vi "Display Album Library.vi"(8 "error in (no error)":errorcluster, 10 "MusicLibrary":refnum<class "MusicLibrary.lvclass">, 11 "SongBrowserActor in":refnum<class "SongBrowserActor.lvclass">) -> (0 "error out":errorcluster, 3 "SongBrowserActor out":refnum<class "SongBrowserActor.lvclass">)   [LabVIEW 2015, in "SongBrowserActor.lvlib" / "SongBrowserActor.lvclass"]
uses:
  SongBrowserActor.lvclass
  file/MusicElement/MusicElementLibrary/MusicLibrary/MusicLibrary.lvclass
  SongBrowserActor.lvclass/SongBrowserActor.ctl
  builds/xctls/Album Browser/Album Browser.lvlibp/app/xctls/Album Browser/Album Browser/Album Browser.xctl
  file/MusicElement/MusicElementLibrary/MusicElementLibrary.lvclass
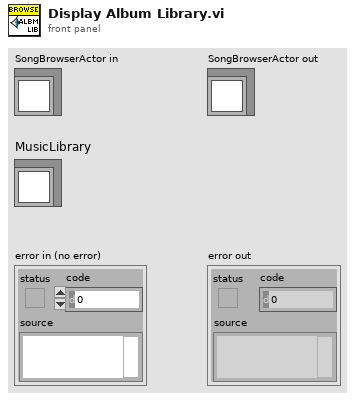
[diagram p1: front panel]
types:
  T1 = typedef "Music Library Element Display.ctl" = cluster{"Name":string, "Details":string, "Duration (s)":T2, "Click":bool}
  T2 = typedef "Song.lvclass/Song Duration.ctl" = timestamp
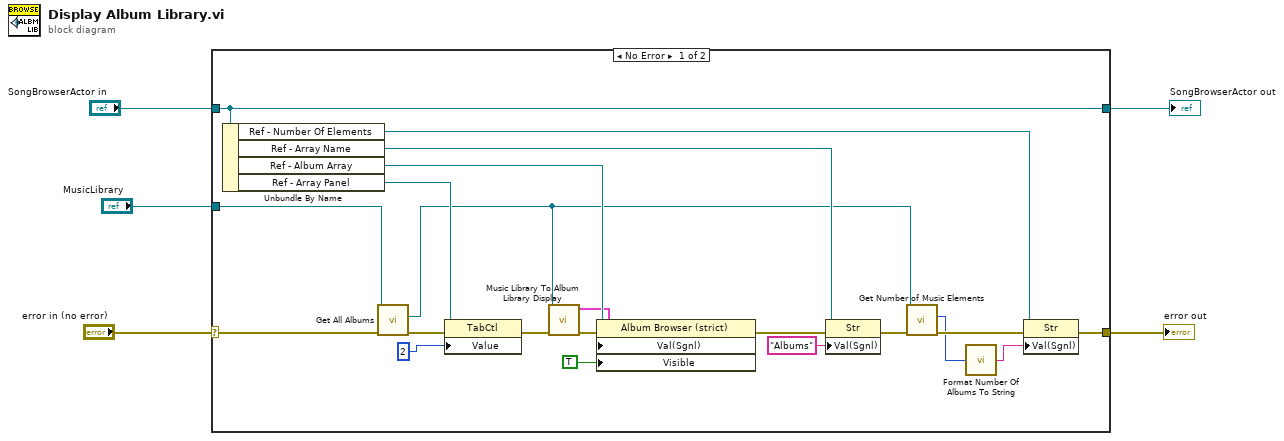
[diagram p0: block diagram]
diagram:
  n1 = case shown="No Error" "error in (no error)" {
    selector: "error in (no error)" -> [w9 w28]
    tunnel: [w17 w28] -> w4
    tunnel: [w26 w27] -> w2
    tunnel: "SongBrowserActor in" -> [w26 w27]
    tunnel: "MusicLibrary" -> [w7 _]
    frame No Error {
      n2 = Unbundle By Name(w26) -> ("Ref - Number Of Elements"=w18:refnum<vi>, "Ref - Array Name"=w20:refnum<vi>, "Ref - Album Array"=w25:refnum<vi>, "Ref - Array Panel"=w14:refnum<vi>)
      n3 = call "Get All Albums.vi"("error in (no error)"=w9, "MusicLibrary in"=w7) -> ("error out"=w8:errorcluster, "MusicLibrary"=w6:refnum<class "MusicLibrary.lvclass">)  [unwired: 7 in, 1 out]
      n4 = property class="TabCtl"(reference=w14, error in=w8, "Value"=2) -> (error out=w15:errorcluster)  [unwired: 1 out]
      n5 = call "Music Library To Album Library Display.vi"("error in (no error)"=w15, "MusicLibrary"=w6) -> ("error out"=w22:errorcluster, "Music Library Display Array"=w23:T1[])  [unwired: 8 in]
      n6 = property class="Album Browser (strict)"(reference=w25, error in=w22, "Val(Sgnl)"=w23, "Visible"=TRUE) -> (error out=w21:errorcluster)  [unwired: 1 out]
      n7 = property class="Str"(reference=w20, error in=w21, "Val(Sgnl)"="Albums" ("Value (Signaling)")) -> (error out=w12:errorcluster)  [unwired: 1 out]
      n8 = call "Get Number of Music Elements.vi"("error in (no error)"=w12, "MusicElementLibrary in"=w6) -> ("error out"=w11:errorcluster, "Size"=w10:i32)  [unwired: 7 in, 1 out]
      n9 = call "Format Number Of Albums To String.vi"("Number Of Songs"=w10) -> ("Formatted"=w16:string)
      n10 = property class="Str"(reference=w18, error in=w11, "Val(Sgnl)"=w16) -> (error out=w17:errorcluster)  [unwired: 1 out]
    }
    frame Error {
    }
  }
  "error out" <- w4
  "SongBrowserActor out" <- w2
